vi "Run.vi"(8 "error in (no error)":errorcluster, 9 "s on last turn":dbl=0.3439976484514773, 10 "Maze (0: Empty, -1: Enemy. >0: Teammate":i32[][](array[numeric])=[[16, 0, 18], [0, 14, 0], [0, 0, 0]], 11 "Mother In":refnum<class "Mother.lvclass">=refnum) -> (0 "error out":errorcluster, 1 "Direction":T1=enum."SE", 2 "Action":T2=enum."Replicate", 3 "Mother Out":refnum<class "Mother.lvclass">, 4 "Replicated":refnum<class "Runner.lvclass">)   [LabVIEW 2014, in "Mother.lvclass"]
uses:
  Mother.lvclass
  Action Enum.ctl
  Direction Enum.ctl
  Runner.lvclass
  Protector/Protector.lvclass
  Queen Bee Steps.ctl
  Mother.lvclass/Mother.ctl
  SquareStatus.ctl
  Attack Options.ctl
  Formic Types.ctl
  SquareBattle.lvclass
panel:
  out "Kam?":bool
  out "Map":i32[](array[numeric])=[16, 0, 18, 0, 0, 0, 0, 0]
  in  "Protectors":i32[](array[numeric])=[2, 6]
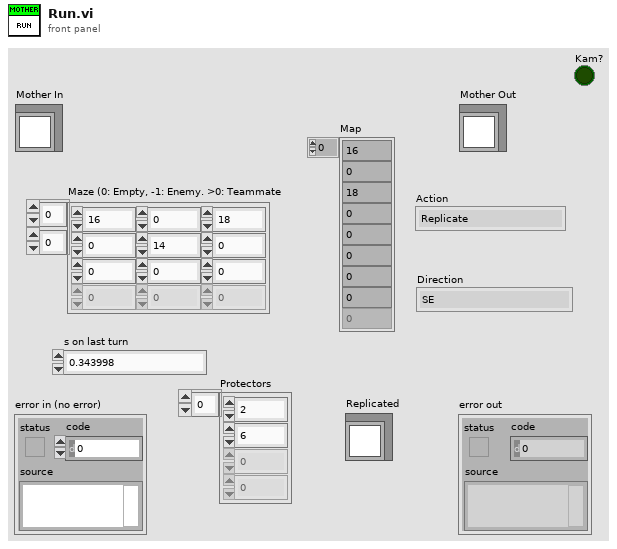
[diagram p1: front panel]
types:
  T1 = typedef "SquareBattle.lvclass/Direction Enum.ctl" = enum16{"NW", "N", "NE", "E", "SE", "S", "SW", "W"}
  T2 = typedef "SquareBattle.lvclass/Action Enum.ctl" = enum16{"Wait", "Move", "Attack", "Replicate"}
  T3 = typedef "Mother.lvclass/Queen Bee Steps.ctl" = enum16{"Attack?", "Migrate?", "Kamikaze?", "Protect?", "Procreate?", "Build Army"}
  T4 = typedef "Mother.lvclass/SquareStatus.ctl" = cluster{"ID":i32, "Heartbeat":bool}
  T5 = typedef "Mother.lvclass/SquareStatus DVR.ctl" = refnum<data-value>
  T6 = typedef "Mother.lvclass/Attack Options.ctl" = enum16{"Attack", "Run", "Distract"}
  T7 = typedef "Mother.lvclass/Formic Types.ctl" = enum16{"Queen Bee", "Protector Bee", "Daughter Bee", "Worker Bee", "Coward"}
  T8 = typedef "Mother.lvclass/Kamikaze DVR.ctl" = refnum<data-value>
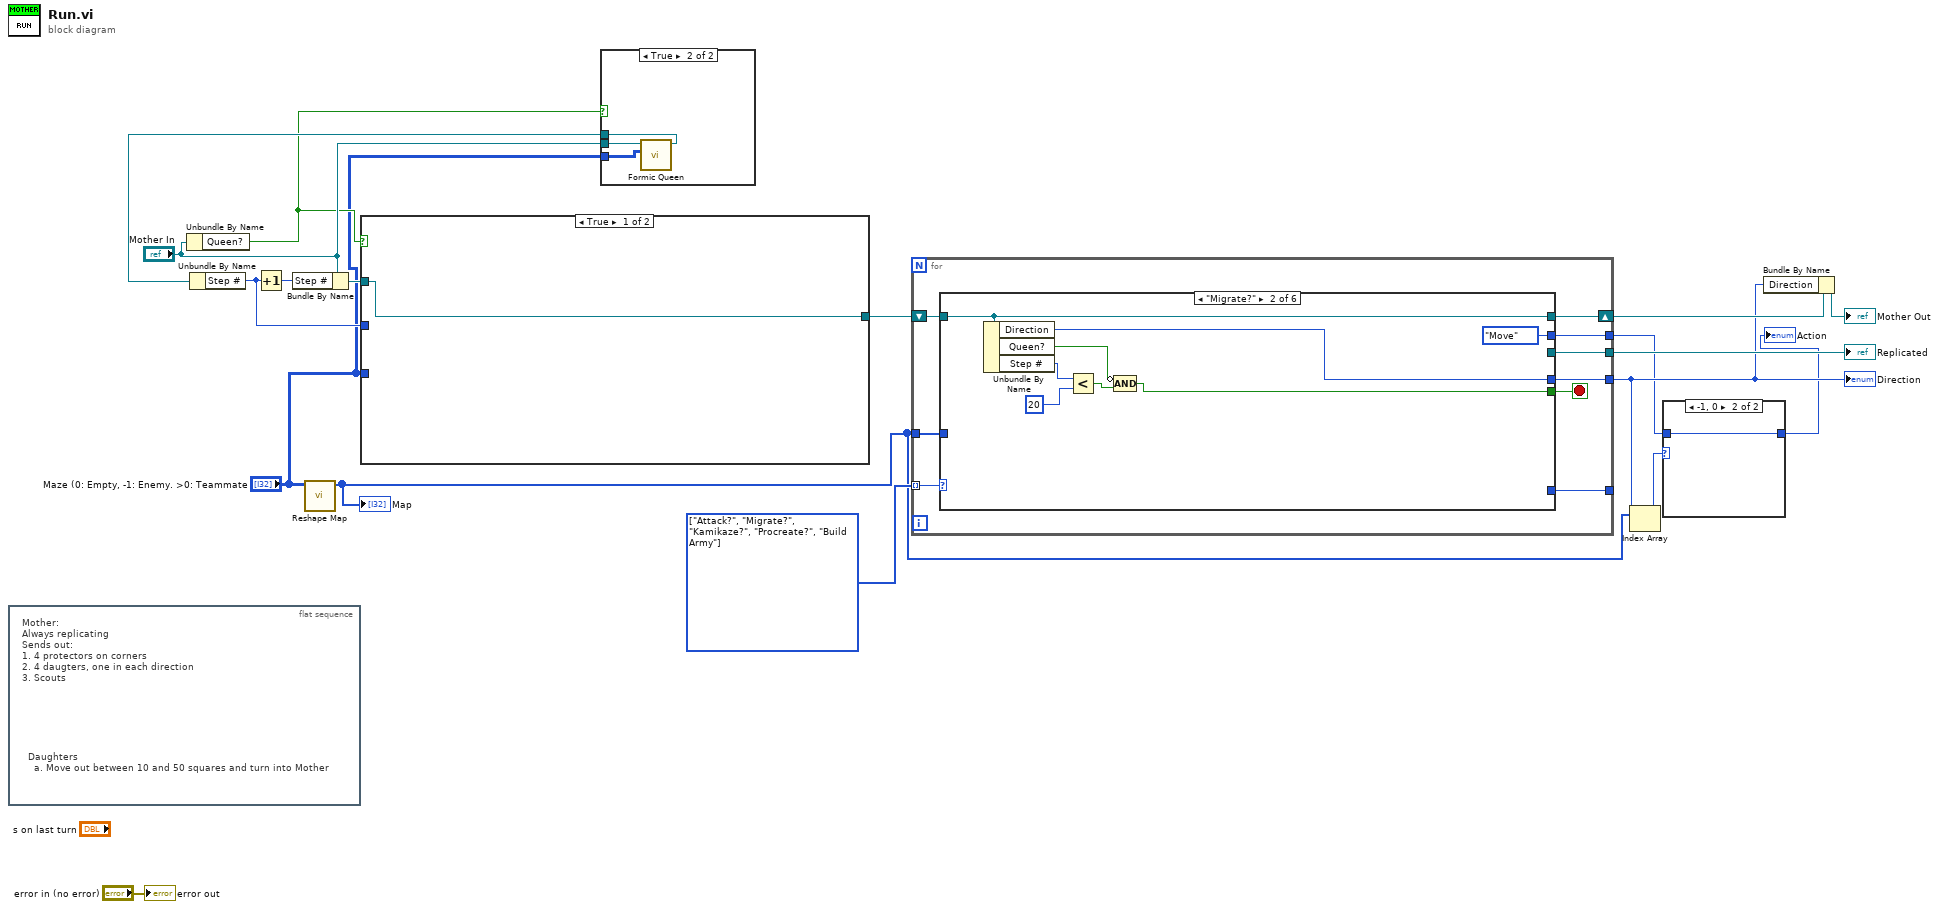
[diagram p0: block diagram]
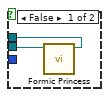
[diagram p2: hidden frame]
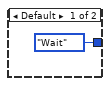
[diagram p3: hidden frame]
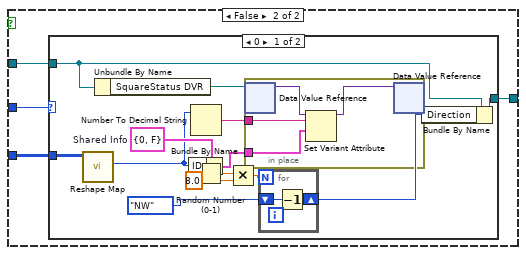
[diagram p4: hidden frame]
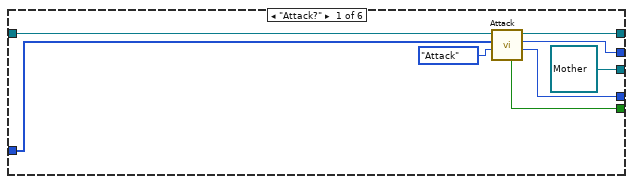
[diagram p6: hidden frame]
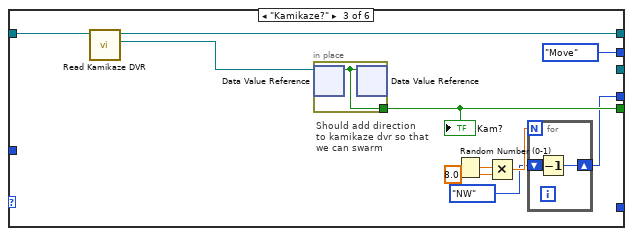
[diagram p7: hidden frame]
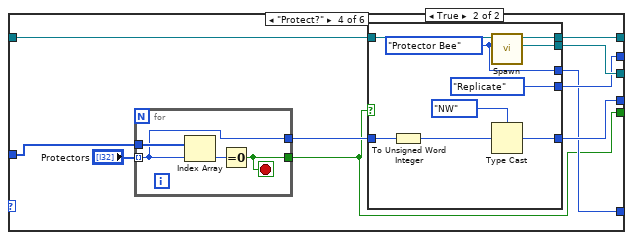
[diagram p8: hidden frame]
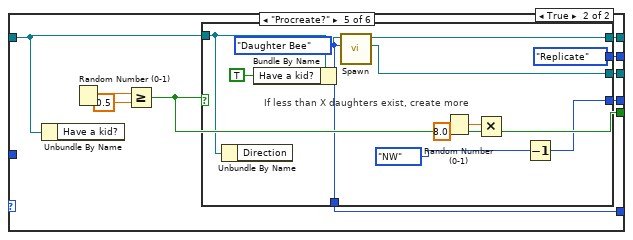
[diagram p10: hidden frame]
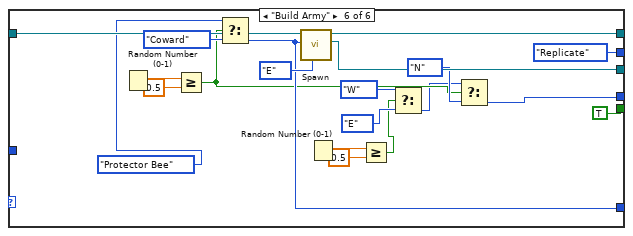
[diagram p12: hidden frame]
diagram:
  w15 = T3[] [enum."Attack?", enum."Migrate?", enum."Kamikaze?", enum."Procreate?", enum."Build Army"] items=["Attack?", "Migrate?", "Kamikaze?", "Protect?", "Procreate?", "Build Army"]
  n1 = flat-sequence {
    frame #0 {
      # "Daughters\n  a. Move out between 10 and 50 squares and turn into Mother"
      # "Mother:\nAlways replicating\nSends out:\n1. 4 protectors on corners\n2. 4 daugters, one in each direction\n3. Scouts"
    }
  }
  n2 = Unbundle By Name("Mother In") -> ("Queen?"=w2:bool)
  n3 = call "Reshape Map.vi"("Maze (0: Empty, -1: Enemy. >0: Teammate"="Maze (0: Empty, -1: Enemy. >0: Teammate") -> ("Map"=w9:i32[])  [unwired: 9 in, 1 out]
  "Map" <- w9
  n4 = case shown="True" w2 {
    tunnel: "Mother In" -> [w20 w23]
    tunnel: [w19 w22] -> w3
    tunnel: "Maze (0: Empty, -1: Enemy. >0: Teammate" -> [_ w21]
    frame False {
      n5 = call "Formic Princess.vi"("Mother in"=w20) -> ("Mother out"=w19:refnum<class "Mother.lvclass">)  [unwired: 9 in, 1 out]
    }
    frame True {
      n6 = call "Formic Queen.vi"("Maze (0: Empty, -1: Enemy. >0: Teammate"=w21, "Mother in"=w23) -> ("Mother out"=w22:refnum<class "Mother.lvclass">)  [unwired: 8 in, 1 out]
    }
  }
  n7 = Unbundle By Name(w3) -> ("Step #"=w14:i32)
  n8 = Increment(x=w14) -> (x+1=w17:i32)
  n9 = Bundle By Name(cluster="Mother In", "Step #"=w17) -> (w13:refnum<class "Mother.lvclass">)
  n10 = case shown="True" w2 {
    tunnel: w13 -> [w24 w27]
    tunnel: [w24 w28] -> w12
    tunnel: w14 -> [_ w26]
    tunnel: "Maze (0: Empty, -1: Enemy. >0: Teammate" -> [_ w25]
    frame True {
    }
    frame False {
      n11 = case shown="0" w26 {
        tunnel: w27 -> [w40 w48]
        tunnel: [w30 w48] -> w28
        tunnel: w25 -> [w35 _]
        frame 0 {
          w39 = T4 {"ID"=0, "Heartbeat"=FALSE}  # Shared Info
          n12 = call "Reshape Map.vi"("Maze (0: Empty, -1: Enemy. >0: Teammate"=w35) -> ("SelfID"=w36:i32)  [unwired: 9 in, 1 out]
          n13 = Unbundle By Name(w40) -> ("SquareStatus DVR"=w41:T5)
          n14 = Bundle By Name(cluster=w39, "ID"=w36) -> (w37:T4)
          n15 = Number To Decimal String(number=w36) -> (decimal integer string=w38:string)  [unwired: 1 in]
          n16 = Random Number (0-1)() -> (number: 0 to 1=w31:dbl)
          n17 = Multiply(x=w31, y=8.0) -> (x*y=w33:dbl)
          n18 = in-place {
            in-place-border: w38 -> [w45]
            in-place-border: w37 -> [w44]
            n19 = in-place-dvr #1(w41) -> (w47:variant)  [unwired: 1 out]
            n20 = Set Variant Attribute(Variant=w47, name=w45, value=w44) -> (Variant out=w46:variant)  [unwired: 1 in, 2 out]
            n21 = in-place-dvr #1(w46) -> ()  [unwired: 2 out]
          }
          n22 = for {
            N: w33 -> [_]
            shift-right: [w42] -> w29
            shift-left: Direction_Enum."NW" ("Direction") -> [w43]
            n23 = Decrement(x=w43) -> (x-1=w42:T1)
          }
          n24 = Bundle By Name(cluster=w40, "Direction"=w29) -> (w30:refnum<class "Mother.lvclass">)
        }
        frame Default {
        }
      }
    }
  }
  n25 = for {
    tunnel: w9 -> [w55]
    shift-right: [w56] -> w16
    shift-left: w12 -> [w57]
    tunnel: [w54] -> w6
    tunnel: [w53] -> w8
    tunnel: w15 -> [w52] mode=indexing
    tunnel: [w50] -> w11
    tunnel: [w49] -> _
    stop <- w51 stop-if-true
    n26 = case shown="\"Migrate?\"" w52 {
      tunnel: w57 -> [w64 w73 w83 w96 w114 w151]
      tunnel: [w63 w73 w80 w95 w117 w148] -> w56
      tunnel: w55 -> [w62 _ _ w92 _ _]
      tunnel: [w61 Action_Enum."Move" ("Action") Action_Enum."Move" ("Action") w93 w119 Action_Enum."Replicate" ("Action")] -> w54
      tunnel: [w60 w66 w74 w89 w118 w139] -> w53
      tunnel: [w59 w68 w81 w87 w111 TRUE ("Enemy Found?")] -> w51
      tunnel: [refnum<class "Mother.lvclass"> refnum ("Replicated") _ _ w94 w116 w147] -> w50
      tunnel: [_ _ _ w88 w115 w141] -> w49
      frame "Attack?" {
        n27 = call "Attack.vi"("Attack?"=Attack_Options."Attack", "Maze (0: Empty, -1: Enemy. >0: Teammate"=w62, "Mother in"=w64) -> ("Direction"=w60:T1, "Action"=w61:T2, "Mother out"=w63:refnum<class "Mother.lvclass">, "Enemy Found?"=w59:bool)  [unwired: 3 in, 2 out]
      }
      frame "Migrate?" {
        n28 = Unbundle By Name(w73) -> ("Direction"=w66:T1, "Queen?"=w72:bool, "Step #"=w71:i32)
        n29 = Less?(x=w71, y=20 ("# Steps")) -> (x < y?=w70:bool)
        n30 = Compound Arithmetic op=AND(invert w72, w70) -> (w68:bool)
      }
      frame "Kamikaze?" {
        # "Should add direction\nto kamikaze dvr so that\nwe can swarm"
        n31 = call "Read Kamikaze DVR.vi"("Mother in"=w83) -> ("Kamikaze DVR"=w79:T8, "Mother out"=w80:refnum<class "Mother.lvclass">)  [unwired: 8 in, 1 out]
        n32 = in-place {
          in-place-border: [w86] -> w81
          n33 = in-place-dvr #2(w79) -> (w86:bool)  [unwired: 1 out]
          n34 = in-place-dvr #2(w86) -> ()  [unwired: 2 out]
        }
        "Kam?" <- w81
        n35 = Random Number (0-1)() -> (number: 0 to 1=w78:dbl)
        n36 = Multiply(x=w78, y=8.0) -> (x*y=w76:dbl)
        n37 = for {
          N: w76 -> [_]
          shift-right: [w85] -> w74
          shift-left: Direction_Enum."NW" ("Direction") -> [w84]
          n38 = Decrement(x=w84) -> (x-1=w85:T1)
        }
      }
      frame "Protect?" {
        n39 = for {
          tunnel: w92 -> [w110]
          tunnel: [w109] -> w87
          tunnel: "Protectors" -> [w107] mode=indexing
          tunnel: [w107] -> w90
          stop <- w109 stop-if-true
          n40 = Index Array(array=w110, index=w107) -> (element=w108:i32)
          n41 = Equal To 0?(x=w108) -> (x = 0?=w109:bool)
        }
        n42 = case shown="True" w87 {
          tunnel: w96 -> [w97 w106]
          tunnel: [w97 w105] -> w95
          tunnel: [_ w104] -> w94
          tunnel: [_ Action_Enum."Replicate" ("Action")] -> w93
          tunnel: w90 -> [_ w101]
          tunnel: [_ w100] -> w89
          tunnel: [_ w98] -> w88
          frame False {
          }
          frame True {
            w98 = Formic_Types."Protector Bee"
            n43 = To Unsigned Word Integer(number=w101) -> (unsigned 16bit integer=w102:u16)
            n44 = call "Spawn.vi"(10:w98, "Mother in"=w106) -> ("Replicated Class"=w104:refnum<class "Mother.lvclass">, "Mother out"=w105:refnum<class "Mother.lvclass">)  [unwired: 7 in, 1 out]
            n45 = Type Cast(type=Direction_Enum."NW" ("Direction"), x=w102) -> (*(type *) &x=w100:T1)
          }
        }
      }
      frame "Procreate?" {
        n46 = Unbundle By Name(w114) -> ()  [unwired: 1 out]
        n47 = Random Number (0-1)() -> (number: 0 to 1=w113:dbl)
        n48 = Greater Or Equal?(x=w113, y=0.5) -> (x >= y?=w111:bool)
        n49 = case shown="True" w111 {
          tunnel: [_ Action_Enum."Replicate" ("Action")] -> w119
          tunnel: [_ w123] -> w118
          tunnel: [w120 w130] -> w117
          tunnel: [_ w129] -> w116
          tunnel: [_ w128] -> w115
          tunnel: w114 -> [w120 w121]
          frame False {
          }
          frame True {
            w128 = Formic_Types."Daughter Bee"
            # "If less than X daughters exist, create more"
            n50 = Unbundle By Name(w121) -> ()  [unwired: 1 out]
            n51 = Bundle By Name(cluster=w121, "Have a kid?"=TRUE) -> (w127:refnum<class "Mother.lvclass">)
            n52 = call "Spawn.vi"(10:w128, "Mother in"=w127) -> ("Replicated Class"=w129:refnum<class "Mother.lvclass">, "Mother out"=w130:refnum<class "Mother.lvclass">)  [unwired: 7 in, 1 out]
            n53 = Random Number (0-1)() -> (number: 0 to 1=w125:dbl)
            n54 = Multiply(x=w125, y=8.0) -> ()  [unwired: 1 out]
            n55 = Decrement(x=Direction_Enum."NW" ("Direction")) -> (x-1=w123:T1)
          }
        }
      }
      frame "Build Army" {
        n56 = Random Number (0-1)() -> (number: 0 to 1=w142:dbl)
        n57 = Greater Or Equal?(x=w142, y=0.5) -> (x >= y?=w137:bool)
        n58 = Select(t=Formic_Types."Protector Bee", s=w137, f=Formic_Types."Coward") -> (s? t:f=w141:T7)
        n59 = call "Spawn.vi"("Start Direction"=Direction_Enum."E", 10:w141, "Mother in"=w151) -> ("Replicated Class"=w147:refnum<class "Mother.lvclass">, "Mother out"=w148:refnum<class "Mother.lvclass">)  [unwired: 6 in, 1 out]
        n60 = Random Number (0-1)() -> (number: 0 to 1=w136:dbl)
        n61 = Greater Or Equal?(x=w136, y=0.5) -> (x >= y?=w132:bool)
        n62 = Select(t=Direction_Enum."W", s=w132, f=Direction_Enum."E" ("Direction")) -> (s? t:f=w134:T1)
        n63 = Select(t=w134, s=w137, f=Direction_Enum."N" ("Direction")) -> (s? t:f=w139:T1)
      }
    }
  }
  "Direction" <- w8
  "Replicated" <- w11
  n64 = Index Array(array=w9, index=w8) -> (element=w7:i32)
  n65 = case shown="-1, 0" w7 {
    tunnel: w6 -> [_ w153]
    tunnel: [Action_Enum."Wait" ("Action") w153] -> w5
    frame Default {
    }
    frame -1, 0 {
    }
  }
  "Action" <- w5
  n66 = Bundle By Name(cluster=w16, "Direction"=w8) -> (→"Mother Out":refnum<class "Mother.lvclass">)
  "error out" <- "error in (no error)"
